vi "ATR latch.vi"(11 "enabled channels":u32) -> (2 "new value":bool, 3 "ATR  out":u8)   [LabVIEW 2023]
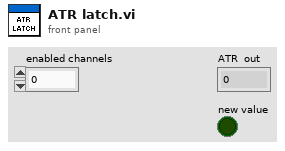
[diagram p1: front panel]
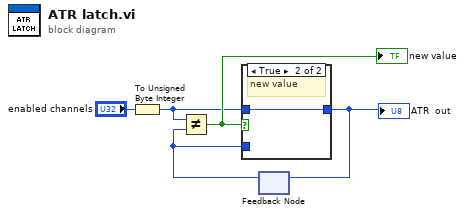
[diagram p0: block diagram]
diagram:
  n1 = To Unsigned Byte Integer(number="enabled channels") -> (unsigned 8bit integer=w1:u8)
  n2 = feedback #1() -> (w4:u8)  [unwired: 1 in]
  n3 = Not Equal?(x=w1, y=w4) -> (x != y?=w2:bool)
  "new value" <- w2
  n4 = case shown="True" w2 {
    tunnel: w1 -> [_ w7]
    tunnel: [w6 w7] -> w3
    tunnel: w4 -> [w6 _]
    frame False {
      # "latched value"
    }
    frame True {
      # "new value"
    }
  }
  "ATR  out" <- w3
  n5 = feedback-in #1(w3) -> ()
